vi "Property Node Type.vi"() -> ()   [LabVIEW 2015]
uses:
  <resource>/objmgr/slsc.rc
panel:
  in  "Cluster":T1
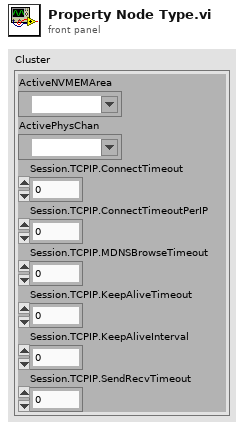
[diagram p1: front panel]
types:
  T1 = cluster{"ActiveNVMEMArea":refnum<k21>, "ActivePhysChan":refnum<k21>, "Session.TCPIP.ConnectTimeout":dbl, "Session.TCPIP.ConnectTimeoutPerIP":dbl, "Session.TCPIP.MDNSBrowseTimeout":dbl, "Session.TCPIP.KeepAliveTimeout":dbl, "Session.TCPIP.KeepAliveInterval":dbl, "Session.TCPIP.SendRecvTimeout":dbl}
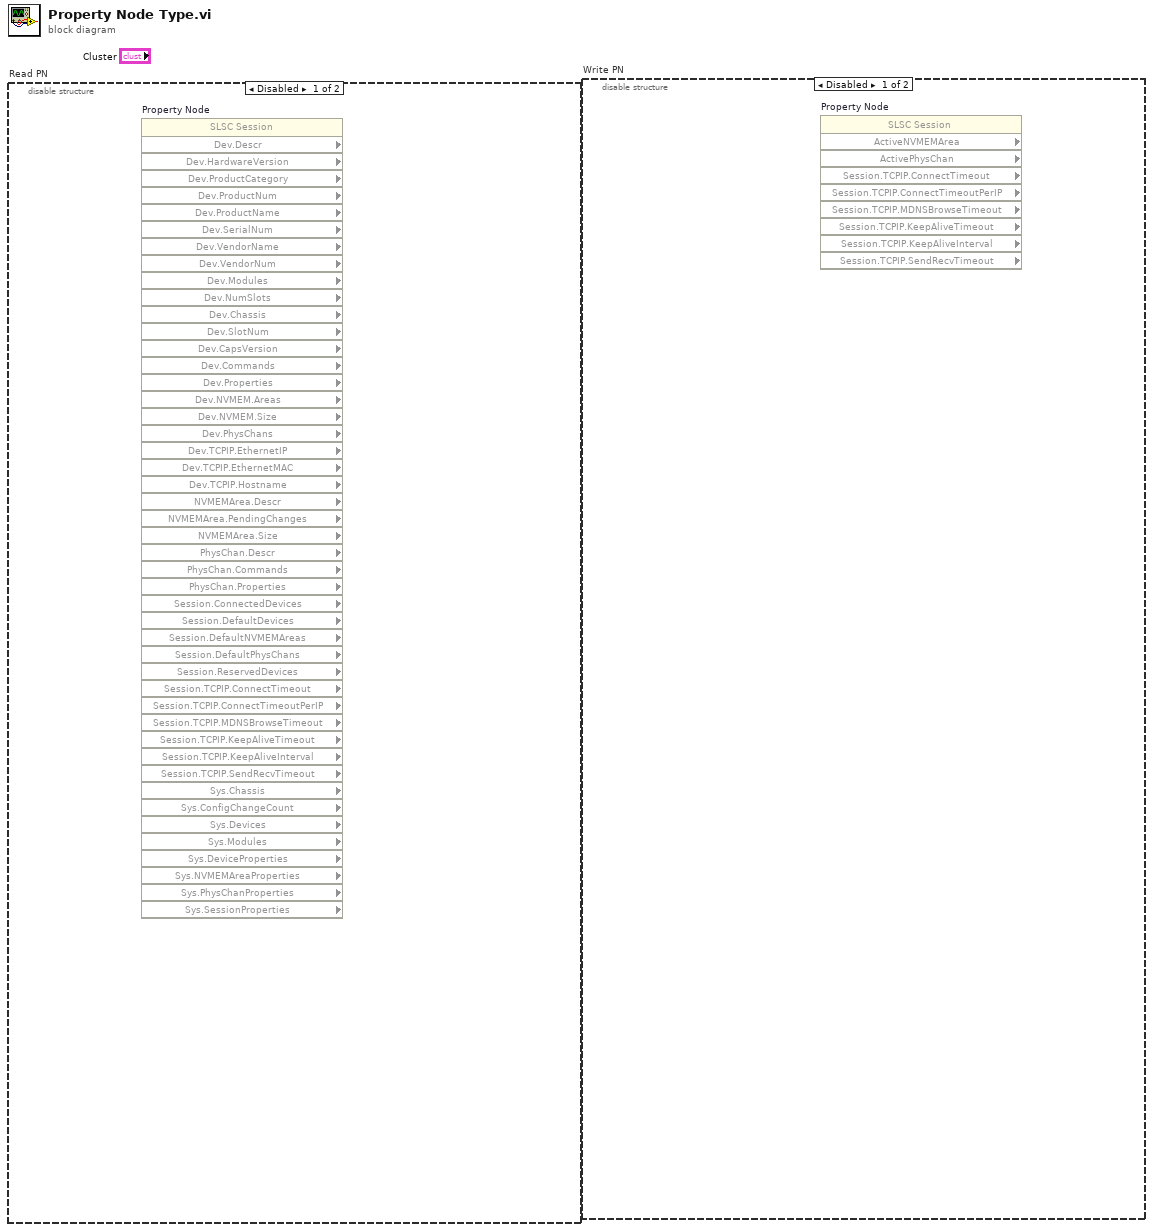
[diagram p0: block diagram]
diagram:
  n1 = disable-structure "Read PN" shown="Disabled" {
    frame Disabled {
      n2 = property on="Property Node" class="SLSC Session"() -> ("Dev.Descr"=w46:string, "Dev.HardwareVersion"=w45:string, "Dev.ProductCategory"=w44:i32, "Dev.ProductNum"=w43:u32, "Dev.ProductName"=w42:string, "Dev.SerialNum"=w41:string, "Dev.VendorName"=w40:string, "Dev.VendorNum"=w39:u32, "Dev.Modules"=w38:refnum<k21>[], "Dev.NumSlots"=w37:u32, "Dev.Chassis"=w36:refnum<k21>, "Dev.SlotNum"=w35:u32, "Dev.CapsVersion"=w34:string, "Dev.Commands"=w33:refnum<k21>[], "Dev.Properties"=w32:refnum<k21>[], "Dev.NVMEM.Areas"=w31:refnum<k21>[], "Dev.NVMEM.Size"=w30:u32, "Dev.PhysChans"=w29:refnum<k21>[], "Dev.TCPIP.EthernetIP"=w28:string, "Dev.TCPIP.EthernetMAC"=w27:string, "Dev.TCPIP.Hostname"=w26:string, "NVMEMArea.Descr"=w25:string, "NVMEMArea.PendingChanges"=w24:bool, "NVMEMArea.Size"=w23:u32, "PhysChan.Descr"=w22:string, "PhysChan.Commands"=w21:refnum<k21>[], "PhysChan.Properties"=w20:refnum<k21>[], "Session.ConnectedDevices"=w19:refnum<k21>[], "Session.DefaultDevices"=w18:refnum<k21>[], "Session.DefaultNVMEMAreas"=w17:refnum<k21>[], "Session.DefaultPhysChans"=w16:refnum<k21>[], "Session.ReservedDevices"=w15:refnum<k21>[], "Session.TCPIP.ConnectTimeout"=w14:dbl, "Session.TCPIP.ConnectTimeoutPerIP"=w13:dbl, "Session.TCPIP.MDNSBrowseTimeout"=w12:dbl, "Session.TCPIP.KeepAliveTimeout"=w11:dbl, "Session.TCPIP.KeepAliveInterval"=w10:dbl, "Session.TCPIP.SendRecvTimeout"=w9:dbl, "Sys.Chassis"=w8:refnum<k21>[], "Sys.ConfigChangeCount"=w7:u64, "Sys.Devices"=w6:refnum<k21>[], "Sys.Modules"=w5:refnum<k21>[], "Sys.DeviceProperties"=w4:refnum<k21>[], "Sys.NVMEMAreaProperties"=w3:refnum<k21>[], "Sys.PhysChanProperties"=w2:refnum<k21>[], "Sys.SessionProperties"=w1:refnum<k21>[])  [unwired: 2 in, 2 out]
    }
    frame Enabled {
    }
  }
  n3 = disable-structure "Write PN" shown="Disabled" {
    frame Disabled {
      n4 = property on="Property Node" class="SLSC Session"() -> ("ActiveNVMEMArea"=w54:refnum<k21>, "ActivePhysChan"=w53:refnum<k21>, "Session.TCPIP.ConnectTimeout"=w52:dbl, "Session.TCPIP.ConnectTimeoutPerIP"=w51:dbl, "Session.TCPIP.MDNSBrowseTimeout"=w50:dbl, "Session.TCPIP.KeepAliveTimeout"=w49:dbl, "Session.TCPIP.KeepAliveInterval"=w48:dbl, "Session.TCPIP.SendRecvTimeout"=w47:dbl)  [unwired: 2 in, 2 out]
    }
    frame Enabled {
    }
  }
